vi "FTW-Container-Initialize.vi"(0 "Container":refnum<class "FTW-Container.lvclass">, 5 "LabVIEW Data Structure":variant, 11 "error in":errorcluster) -> (4 "Container out":refnum<class "FTW-Container.lvclass">, 15 "error out":errorcluster)   [LabVIEW 2012, in "FTW-Container.lvclass"]
uses:
  FTW-Container.lvclass
  FTW-Container.lvclass/FTW-Container.ctl
  Error/FTW-ERR-ThrowError.vi
panel:
  # "Inputs"
  # "Outputs"
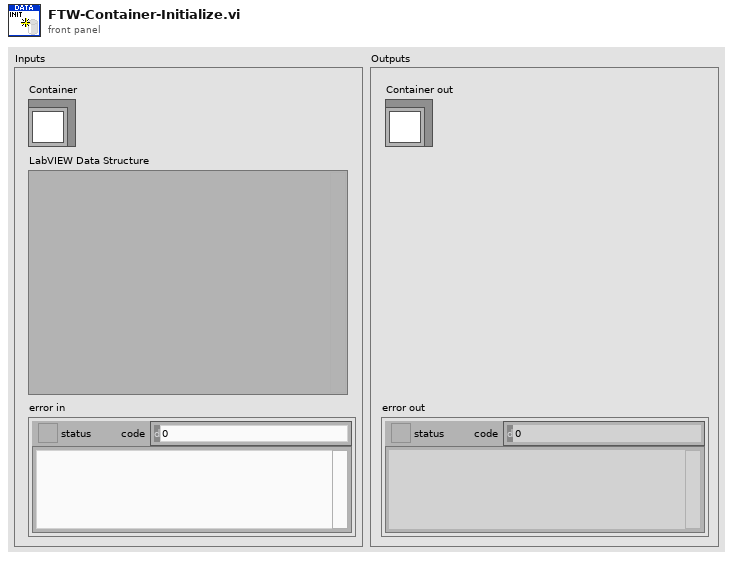
[diagram p1: front panel]
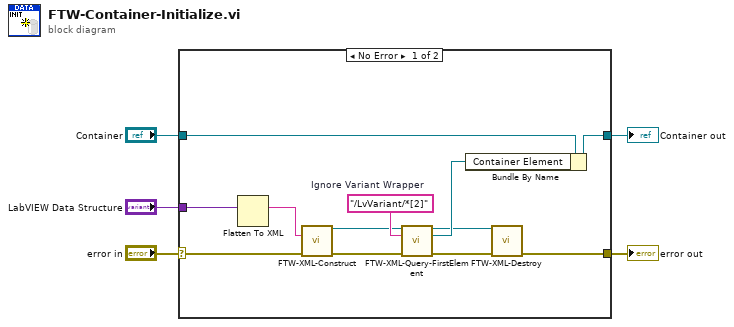
[diagram p0: block diagram]
diagram:
  n1 = case shown="No Error" "error in" {
    selector: "error in" -> [w17 w19]
    tunnel: [w6 w19] -> w5
    tunnel: [w14 w18] -> w1
    tunnel: "Container" -> [w15 w18]
    tunnel: "LabVIEW Data Structure" -> [w16 _]
    frame No Error {
      w12 = "/LvVariant/*[2]"  # Ignore Variant Wrapper
      n2 = Flatten To XML(anything=w16) -> (xml string=w13:string)
      n3 = call "FTW-XML-Construct.vi"("XML String"=w13, "error in"=w17) -> ("XML Document"=w11:refnum<k20>, "error out"=w10:errorcluster)  [unwired: 12 in]
      n4 = call "FTW-XML-Query-FirstElement.vi"("XML Node"=w11, "XPath Query"=w12, "error in"=w10) -> ("XML Node out"=w8:refnum<k20>, "First Matched Element"=w9:refnum<k20>, "error out"=w7:errorcluster)  [unwired: 8 in, 2 out]
      n5 = Bundle By Name(cluster=w15, "Container Element"=w9) -> (w14:refnum<class "FTW-Container.lvclass">)
      n6 = call "FTW-XML-Destroy.vi"("XML Node"=w8, "error in"=w7) -> ("error out"=w6:errorcluster)  [unwired: 13 in]
    }
    frame Error {
    }
  }
  "error out" <- w5
  "Container out" <- w1
